vi "Main.vi"(11 "Module Admin":refnum<class "Delacor_lib_QMH_Module Admin.lvclass">) -> ()   [LabVIEW 2022 SP3, in "HW-201 Manager.lvlib"]
doc: "This template is based off of the Queued Message Handler design pattern and the Queued Message Handler project template that ships with LabVIEW.\n\nThe main difference is that the queue is private to this module and communication between modules is performed via Broadcast and Request events.\n\nRequest events are wrapped in public API methods and are handled in the Event Handling Loop (EHL) of this VI. Any module can register for Broadcast events sent by this module. The EHL generates messages based on user interface actions.\n\nThe Message Handling Loop (MHL) processes messages generated by the EHL, or by other messages. The messages are string values, so new messages can be added easily to the Message Cases case structure in the MHL. Each message cluster can also provide an optional value for Message Data, which is a variant that can be converted to whatever message-specific data is required.\n_____\nBased on DQMH Project Template 7.0.1.1316."
uses:
  HW-201 Manager.lvlib
  <vilib>/Delacor/Delacor QMH/Libraries/Module Admin_class/Delacor_lib_QMH_Module Admin.lvclass
  Module Data--cluster.ctl
  Do Something Argument--cluster.ctl
  <vilib>/Delacor/Delacor QMH/Libraries/Message Queue_class/Delacor_lib_QMH_Message Queue.lvclass/Delacor_lib_QMH_Message Queue.ctl
  Do Something Else Argument--cluster.ctl
  Do Something Else and Wait for Reply Argument--cluster.ctl
  Do Something Else and Wait (Reply Payload)--cluster.ctl
  Stop Argument--cluster.ctl
  <vilib>/Delacor/Delacor QMH/Libraries/Module Admin_class/Delacor_lib_QMH_Module Admin.lvclass/Delacor_lib_QMH_Module Admin.ctl
  <vilib>/Utility/miscctls.llb/LVPointTypeDef.ctl
  <vilib>/Delacor/Delacor QMH/Libraries/Message Queue_class/Delacor_lib_QMH_Enqueue Message (Single).vi
  <vilib>/Delacor/Delacor QMH/Libraries/Module Admin_class/Delacor_lib_QMH_Get External Launch.vi
  <vilib>/Delacor/Delacor QMH/Libraries/Message Queue_class/Delacor_lib_QMH_Message Queue.lvclass
panel:
  out "error out":errorcluster
  out "X":dbl
  out "Status":string
  in  "Simulate MHL Error":bool
  in  "Simulate EHL Error":bool
  in  "Do Something Else <Replace Me>":bool
  in  "Do Something <Replace Me>":bool
  # "These controls have associated \"Value Changed\" events configured in the Event Structure on the diagram.\n\nReplace them (and reconfigure the Event Structure) with the controls you need for your application. \n\nOther processes communicate with this Module via its Public API (wrappers for its Request Events).\n\nThis Module communicates with other processes via its Broadcast Events.\nAny process that wants to receive these messages can register for this module's Broadcast events."
  # "This template is for the DQMH framework. See the block diagram for more information on how to use this template."
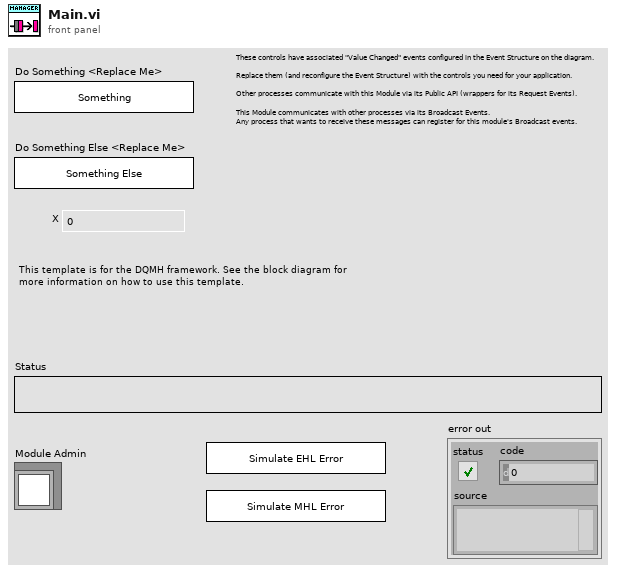
[diagram p1: front panel]
types:
  T1 = typedef "HW-201 Manager.lvlib/Request Events--cluster.ctl" = cluster{"Stop Module":refnum<user-event>, "Do Something":refnum<user-event>, "Do Something Else":refnum<user-event>, "Do Something Else and Wait for Reply":refnum<user-event>, "Show Panel":refnum<user-event>, "Hide Panel":refnum<user-event>, "Get Module Execution Status":refnum<user-event>, "Show Diagram":refnum<user-event>}
  T2 = typedef "HW-201 Manager.lvlib/Module Data--cluster.ctl" = cluster{"Status":string}
  T3 = typedef "HW-201 Manager.lvlib/Do Something Argument--cluster.ctl" = cluster{"Do Something Msg":string}
  T4 = typedef "HW-201 Manager.lvlib/Do Something Else Argument--cluster.ctl" = cluster{"Do Something Else Msg":string, "X":dbl}
  T5 = typedef "HW-201 Manager.lvlib/Do Something Else and Wait for Reply Argument--cluster.ctl" = cluster{"Do Something Else Msg":string, "X":dbl, "Wait Notifier":refnum<notifier>, "wait for reply":bool}
  T6 = enum32{"invalid lock state", "Not Locked", "Locked (No Password)", "Password-protected"}
  T7 = typedef "HW-201 Manager.lvlib/Stop Argument--cluster.ctl" = cluster{"Origin":string, "Exit via Stop Module Req?":bool, "Wait for Module to stop?":bool}
  T8 = typedef "LVPointTypeDef.ctl" = cluster{"Horizontal":i16, "Vertical":i16}
  T9 = enum32{"Invalid", "Standard", "Closed", "Hidden", "Minimized", "Maximized"}
  T10 = typedef "HW-201 Manager.lvlib/Do Something Else and Wait (Reply Payload)--cluster.ctl" = cluster{"Value":dbl, "error":errorcluster}
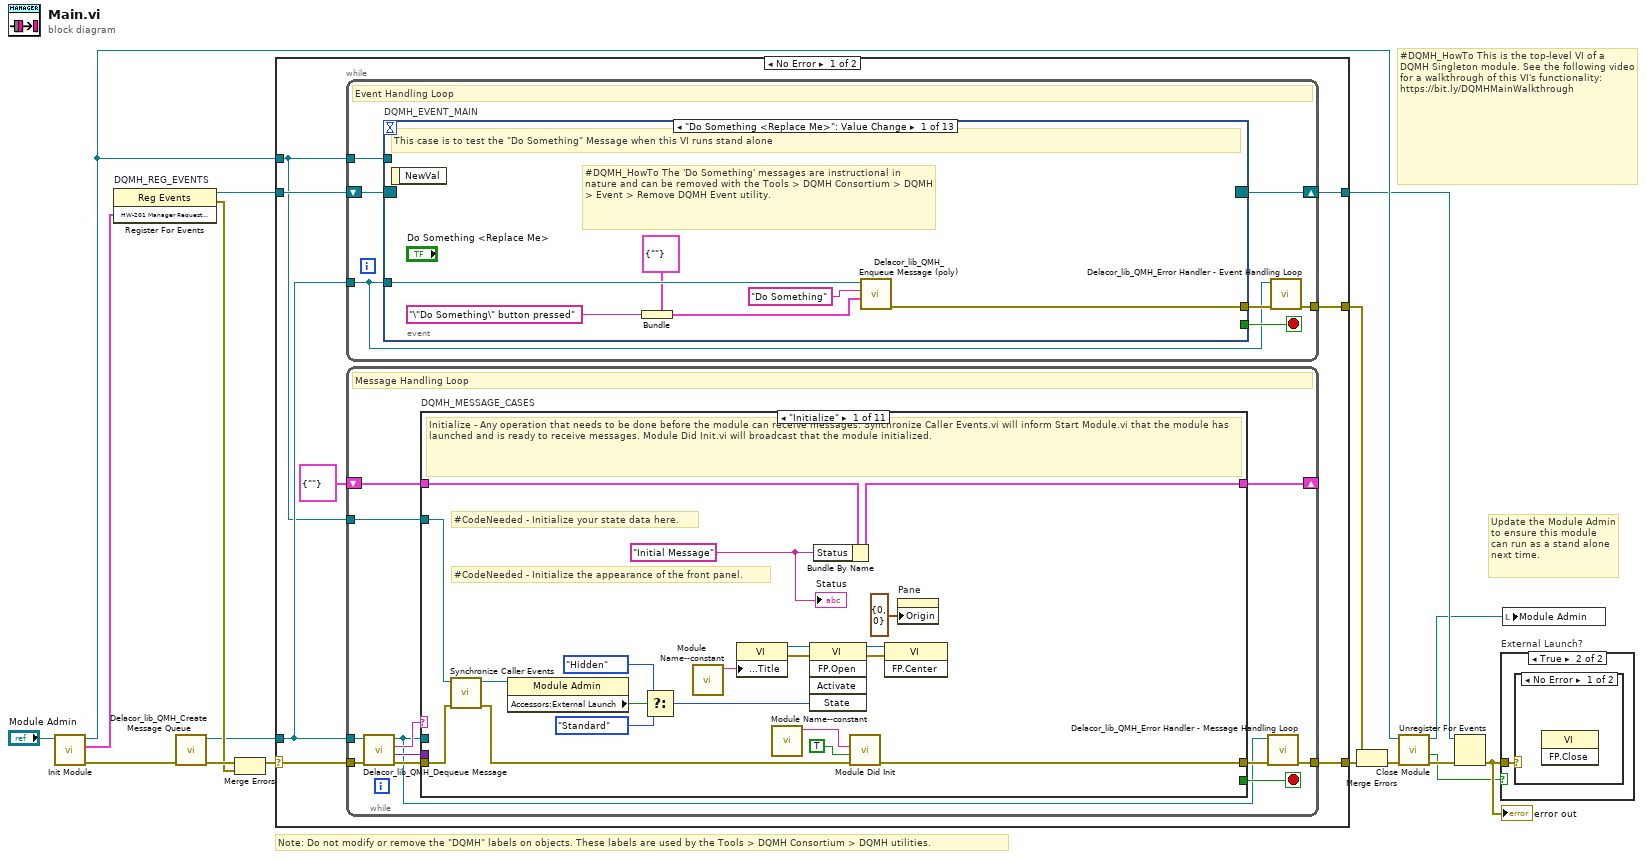
[diagram p0: block diagram]
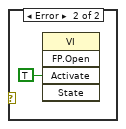
[diagram p3: hidden frame]
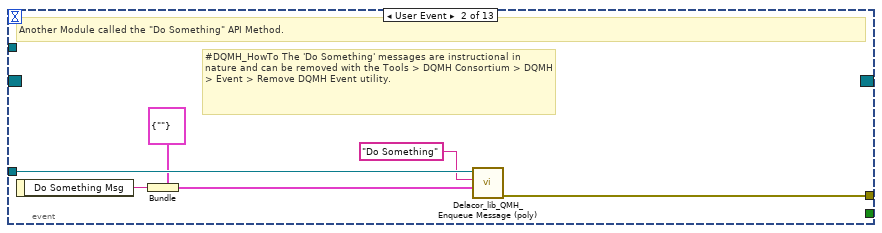
[diagram p4: hidden frame]
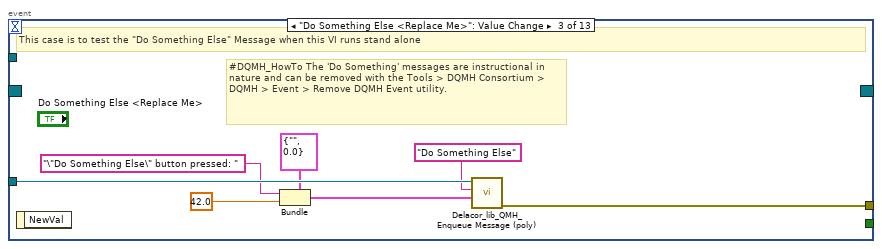
[diagram p5: hidden frame]
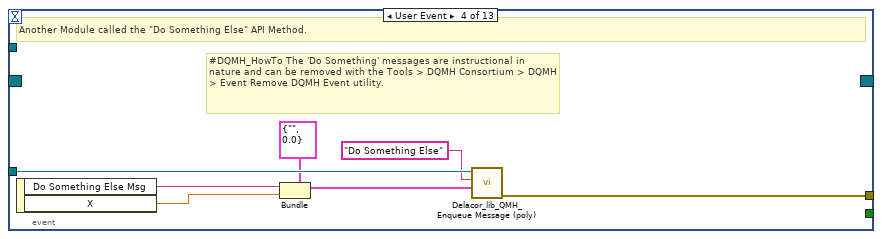
[diagram p6: hidden frame]
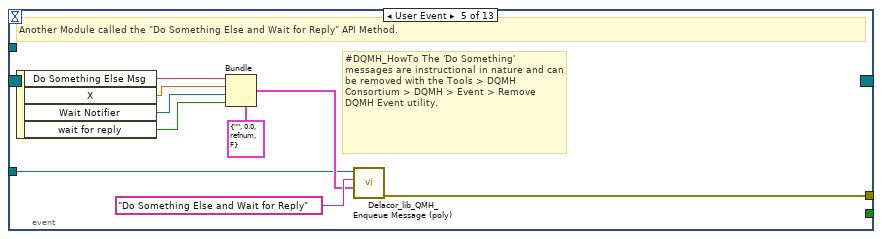
[diagram p7: hidden frame]
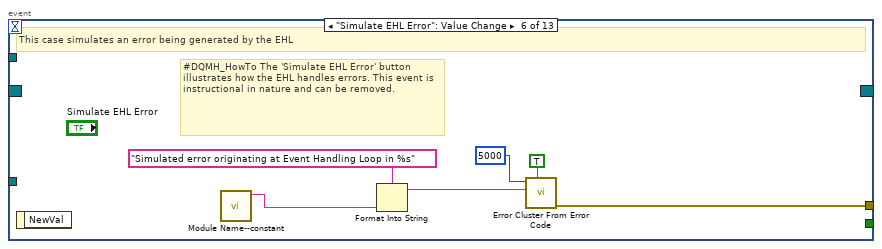
[diagram p8: hidden frame]
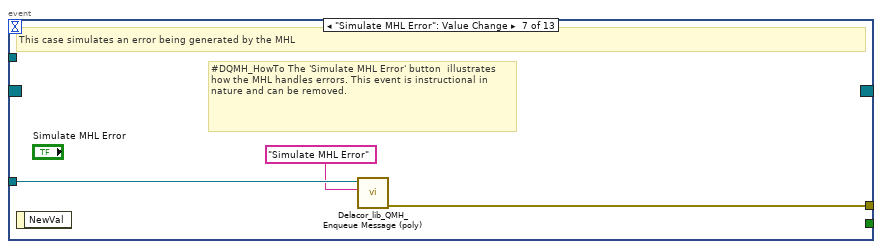
[diagram p9: hidden frame]
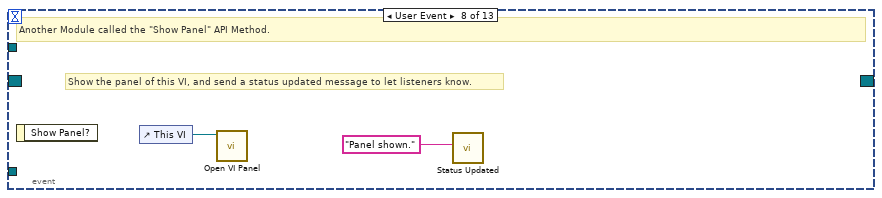
[diagram p10: hidden frame]
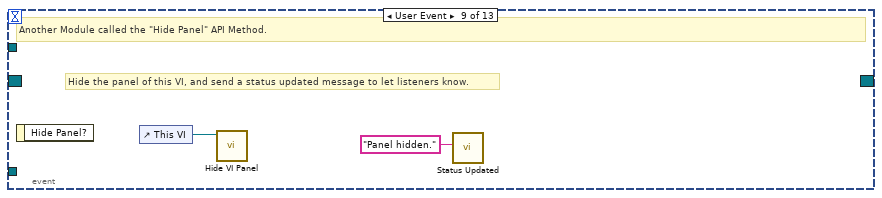
[diagram p11: hidden frame]
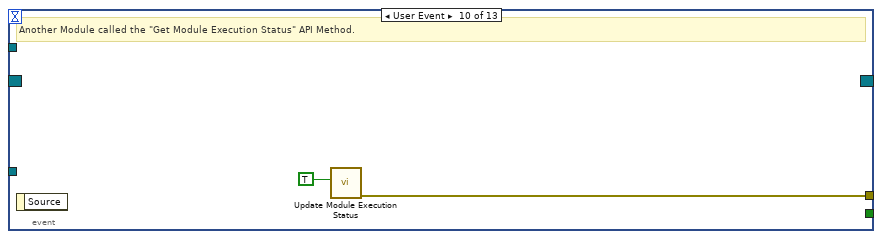
[diagram p12: hidden frame]
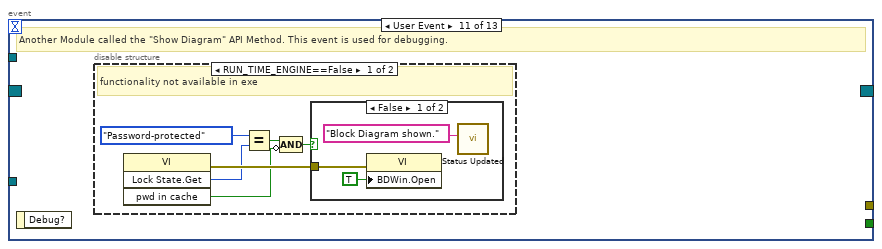
[diagram p13: hidden frame]
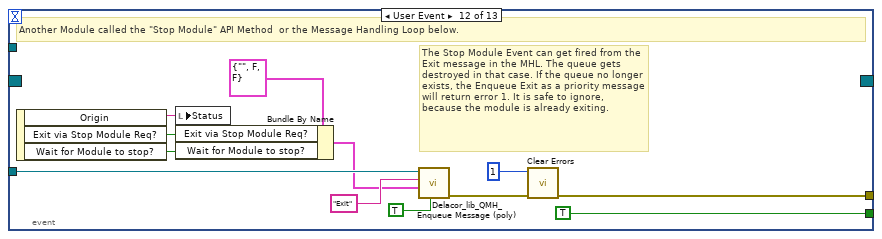
[diagram p16: hidden frame]
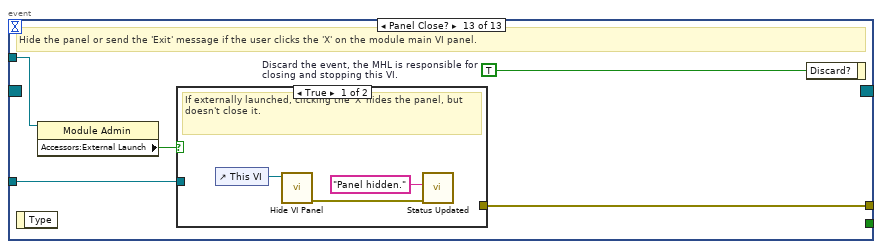
[diagram p17: hidden frame]
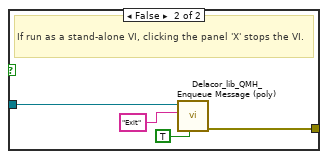
[diagram p18: hidden frame]
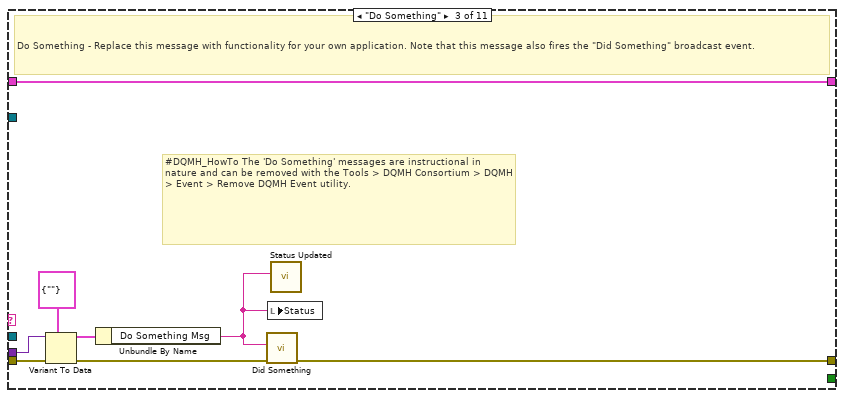
[diagram p20: hidden frame]
diagram:
  # "#DQMH_HowTo This is the top-level VI of a DQMH Singleton module. See the following video for a walkthrough of this VI's functionality: https://bit.ly/DQMHMainWalkthrough"
  # "Note: Do not modify or remove the \"DQMH\" labels on objects. These labels are used by the Tools > DQMH Consortium > DQMH utilities."
  # "Update the Module Admin to ensure this module can run as a stand alone next time."
  n1 = call "Init Module.vi"("Singleton Module Admin in"="Module Admin") -> ("error out"=w16:errorcluster, "HW-201 Manager Request Events"=w5:T1, "Singleton Module Admin out"=w8:refnum<class "Delacor_lib_QMH_Module Admin.lvclass">)  [unwired: 8 in]
  n2 = register-events "DQMH_REG_EVENTS"(w5) -> (reference out=w6:refnum<event-registration>, error out=w9:errorcluster)  [unwired: 2 in]
  n3 = call <vilib>:"Delacor_lib_QMH_Create Message Queue.vi"("error in"=w16) -> ("error out"=w11:errorcluster, "Message Queue"=w4:refnum<class "Delacor_lib_QMH_Message Queue.lvclass">)  [unwired: 9 in]
  n4 = Merge Errors(w11, w9) -> (w10:errorcluster)
  n5 = case shown="No Error" w10 {
    selector: w10 -> [w23 w259]
    tunnel: [w25 w258] -> w17
    tunnel: [w22 w257] -> w7
    tunnel: w6 -> [w20 w257]
    tunnel: w4 -> [w19 w252]
    tunnel: [w24 _] -> w14
    tunnel: w8 -> [w18 w253]
    frame No Error {
      n6 = while {
        tunnel: w19 -> [w26]
        shift-right: [w29] -> w22
        shift-left: w20 -> [w30]
        tunnel: [w31] -> w24
        tunnel: w18 -> [w27]
        stop <- w28 stop-if-true
        # "Event Handling Loop"
        n7 = event "DQMH_EVENT_MAIN" shown="[0] \"Do Something <Replace Me>\": Value Change" {
          selector: w30 -> [_ _ _ _ _ _ _ _ _ _ _ _ _]
          dyn-events: [_ _ _ _ _ _ _ _ _ _ _ _ _] -> w29
          timeout: _ -> [_ _ _ _ _ _ _ _ _ _ _ _ _]
          tunnel: [_ _ _ _ _ _ _ _ _ _ _ TRUE ("Discard?") _] -> w28
          tunnel: w26 -> [w37 w43 w50 w57 w60 _ w75 _ _ _ _ w99 w106]
          tunnel: [w38 w44 w51 w58 w67 w73 w76 _ _ w82 _ w102 w108] -> w32
          tunnel: w27 -> [_ _ _ _ _ _ _ _ _ _ _ _ w105]
          event "Do Something <Replace Me>": Value Change {
            # "#DQMH_HowTo The 'Do Something' messages are instructional in nature and can be removed with the Tools > DQMH Consortium > DQMH > Event > Remove DQMH Event utility."
            # "This case is to test the \"Do Something\" Message when this VI runs stand alone"
            n8 = event-data() -> ()  [unwired: 1 in, 1 out]
            n9 = Bundle(cluster=T3 {"Do Something Msg"=""} ("Do Something Argument"), "Do Something Msg"="\"Do Something\" button pressed" ("\"Do Something\" button pressed")) -> (w33:T3)
            n10 = call-poly <vilib>:"Delacor_lib_QMH_Enqueue Message (poly).vi"("Message Data"=w33, "Message"="Do Something", "Message Queue in"=w37) -> ("error out"=w38:errorcluster)  [unwired: 7 in, 1 out]
          }
          event User Event {
            # "#DQMH_HowTo The 'Do Something' messages are instructional in nature and can be removed with the Tools > DQMH Consortium > DQMH > Event > Remove DQMH Event utility."
            # "Another Module called the \"Do Something\" API Method."
            n11 = event-data() -> ("Do Something Msg"=w40:string)  [unwired: 1 in]
            n12 = Bundle(cluster=T3 {"Do Something Msg"=""} ("Do Something Argument"), "Do Something Msg"=w40) -> (w39:T3)
            n13 = call-poly <vilib>:"Delacor_lib_QMH_Enqueue Message (poly).vi"("Message Data"=w39, "Message"="Do Something", "Message Queue in"=w43) -> ("error out"=w44:errorcluster)  [unwired: 7 in, 1 out]
          }
          event "Do Something Else <Replace Me>": Value Change {
            # "#DQMH_HowTo The 'Do Something' messages are instructional in nature and can be removed with the Tools > DQMH Consortium > DQMH > Event > Remove DQMH Event utility."
            # "This case is to test the \"Do Something Else\" Message when this VI runs stand alone"
            n14 = event-data() -> ()  [unwired: 1 in, 1 out]
            n15 = Bundle(cluster=T4 {"Do Something Else Msg"="", "X"=0.0} ("Do Something Else Argument"), "Do Something Else Msg"="\"Do Something Else\" button pressed: " ("\"Do Something Else\" button pressed"), "X"=42.0) -> (w47:T4)
            n16 = call-poly <vilib>:"Delacor_lib_QMH_Enqueue Message (poly).vi"("Message Data"=w47, "Message"="Do Something Else", "Message Queue in"=w50) -> ("error out"=w51:errorcluster)  [unwired: 7 in, 1 out]
          }
          event User Event {
            # "#DQMH_HowTo The 'Do Something' messages are instructional in nature and can be removed with the Tools > DQMH Consortium > DQMH > Event Remove DQMH Event utility."
            # "Another Module called the \"Do Something Else\" API Method."
            n17 = event-data() -> ("Do Something Else Msg"=w53:string, "X"=w52:dbl)  [unwired: 1 in]
            n18 = Bundle(cluster=T4 {"Do Something Else Msg"="", "X"=0.0} ("Do Something Else Argument"), "Do Something Else Msg"=w53, "X"=w52) -> (w54:T4)
            n19 = call-poly <vilib>:"Delacor_lib_QMH_Enqueue Message (poly).vi"("Message Data"=w54, "Message"="Do Something Else", "Message Queue in"=w57) -> ("error out"=w58:errorcluster)  [unwired: 7 in, 1 out]
          }
          event User Event {
            # "#DQMH_HowTo The 'Do Something' messages are instructional in nature and can be removed with the Tools > DQMH Consortium > DQMH > Event > Remove DQMH Event utility."
            # "Another Module called the \"Do Something Else and Wait for Reply\" API Method."
            n20 = event-data() -> ("Do Something Else Msg"=w63:string, "X"=w62:dbl, "Wait Notifier"=w61:refnum<notifier>, "wait for reply"=w59:bool)  [unwired: 1 in]
            n21 = Bundle(cluster=T5 {"Do Something Else Msg"="", "X"=0.0, "Wait Notifier"=refnum, "wait for reply"=FALSE} ("Do Something Else and Wait for Reply Argument"), "Do Something Else Msg"=w63, "X"=w62, "Wait Notifier"=w61, "wait for reply"=w59) -> (w64:T5)
            n22 = call-poly <vilib>:"Delacor_lib_QMH_Enqueue Message (poly).vi"("Message Data"=w64, "Message"="Do Something Else and Wait for Reply", "Message Queue in"=w60) -> ("error out"=w67:errorcluster)  [unwired: 7 in, 1 out]
          }
          event "Simulate EHL Error": Value Change {
            # "#DQMH_HowTo The 'Simulate EHL Error' button  illustrates how the EHL handles errors. This event is instructional in nature and can be removed."
            # "This case simulates an error being generated by the EHL"
            n23 = event-data() -> ()  [unwired: 1 in, 1 out]
            n24 = call "Module Name--constant.vi"() -> ("Module Name"=w70:string)  [unwired: 11 in]
            n25 = Format Into String(format string="Simulated error originating at Event Handling Loop in %s", w70) -> (resulting string=w71:string)  [unwired: 2 in, 1 out]
            n26 = call <vilib>:"Error Cluster From Error Code.vi"("show call chain? (False)"=TRUE, "error message (\"\")"=w71, "error code (0)"=5000) -> ("error out"=w73:errorcluster)  [unwired: 6 in]
          }
          event "Simulate MHL Error": Value Change {
            # "#DQMH_HowTo The 'Simulate MHL Error' button  illustrates how the MHL handles errors. This event is instructional in nature and can be removed."
            # "This case simulates an error being generated by the MHL"
            n27 = event-data() -> ()  [unwired: 1 in, 1 out]
            n28 = call-poly <vilib>:"Delacor_lib_QMH_Enqueue Message (poly).vi"("Message"="Simulate MHL Error", "Message Queue in"=w75) -> ("error out"=w76:errorcluster)  [unwired: 8 in, 1 out]
          }
          event User Event {
            # "Show the panel of this VI, and send a status updated message to let listeners know."
            # "Another Module called the \"Show Panel\" API Method."
            n29 = event-data() -> ()  [unwired: 1 in, 1 out]
            n30 = control-ref of="This VI"() -> (w78:refnum<vi>)
            n31 = call "Open VI Panel.vi"("VI"=w78) -> ()  [unwired: 10 in, 1 out]
            n32 = call "Status Updated.vi"("Status"="Panel shown." ("format string")) -> ()  [unwired: 10 in, 1 out]
          }
          event User Event {
            # "Hide the panel of this VI, and send a status updated message to let listeners know."
            # "Another Module called the \"Hide Panel\" API Method."
            n33 = event-data() -> ()  [unwired: 1 in, 1 out]
            n34 = control-ref of="This VI"() -> (w80:refnum<vi>)
            n35 = call "Hide VI Panel.vi"("VI"=w80) -> ()  [unwired: 10 in, 1 out]
            n36 = call "Status Updated.vi"("Status"="Panel hidden." ("format string")) -> ()  [unwired: 10 in, 1 out]
          }
          event User Event {
            # "Another Module called the \"Get Module Execution Status\" API Method."
            n37 = event-data() -> ()  [unwired: 1 in, 1 out]
            n38 = call "Update Module Execution Status.vi"("Running?"=TRUE) -> ("error out"=w82:errorcluster)  [unwired: 10 in]
          }
          event User Event {
            # "Another Module called the \"Show Diagram\" API Method. This event is used for debugging."
            n39 = event-data() -> ()  [unwired: 1 in, 1 out]
            n40 = disable-structure shown="RUN_TIME_ENGINE==False" {
              frame condition #0 (active) {
                # "functionality not available in exe"
                n41 = invoke on="Invoke Node" class="VI" method="Lock State.Get"() -> (error out=w88:errorcluster, "Get Lock State"=w87:T6, "pwd in cache"=w84:bool)  [unwired: 4 in, 1 out]
                n42 = Equal?(x=T6."Password-protected", y=w87) -> (x = y?=w85:bool)
                n43 = Compound Arithmetic op=AND(w85, invert w84) -> (w83:bool)
                n44 = case shown="False" w83 {
                  tunnel: w88 -> [w91 _]
                  frame False {
                    n45 = property on="Property Node" class="VI"(error in=w91, "BDWin.Open"=TRUE ("Block Diagram Window:Open")) -> ()  [unwired: 1 in, 2 out]
                    n46 = call "Status Updated.vi"("Status"="Block Diagram shown." ("format string")) -> ()  [unwired: 10 in, 1 out]
                  }
                  frame True {
                    # "Password-protected VI, and the password is not in the cache. Do not show the diagram."
                  }
                }
              }
              frame condition #1 {
              }
            }
          }
          event User Event {
            # "The Stop Module Event can get fired from the Exit message in the MHL. The queue gets destroyed in that case. If the queue no longer exists, the Enqueue Exit as a priority message will return error 1. It is safe to ignore, because the module is already exiting."
            # "Another Module called the \"Stop Module\" API Method  or the Message Handling Loop below."
            n47 = event-data() -> ("Origin"=w98:string, "Exit via Stop Module Req?"=w94:bool, "Wait for Module to stop?"=w93:bool)  [unwired: 1 in]
            n48 = local write "Status"(w98) -> ()
            n49 = Bundle By Name(cluster=T7 {"Origin"="", "Exit via Stop Module Req?"=FALSE, "Wait for Module to stop?"=FALSE} ("Stop Argument"), "Exit via Stop Module Req?"=w94, "Wait for Module to stop?"=w93) -> (w92:T7)
            n50 = call-poly <vilib>:"Delacor_lib_QMH_Enqueue Message (poly).vi"("Priority Message? (F)"=TRUE, "Message Data"=w92, "Message"="Exit", "Message Queue in"=w99) -> ("error out"=w103:errorcluster)  [unwired: 6 in, 1 out]
            n51 = call <vilib>:"Clear Errors.vi"("error in (no error)"=w103, "specific error code to clear (0: all)"=1) -> ("error out"=w102:errorcluster)  [unwired: 4 in, 1 out]
          }
          event Panel Close? {
            w107 = TRUE  # Discard the event, the MHL is responsible for closing and stopping this VI.
            # "Hide the panel or send the 'Exit' message if the user clicks the 'X' on the module main VI panel."
            n52 = event-data() -> ()  [unwired: 1 in, 1 out]
            n53 = property on="Property Node" class="Module Admin"(reference=w105) -> ("Accessors:External Launch"=w104:bool)  [unwired: 1 in, 2 out]
            n54 = case shown="True" w104 {
              tunnel: w106 -> [_ w114]
              tunnel: [_ w115] -> w108
              frame True {
                # "If externally launched, clicking the 'X' hides the panel, but doesn't close it."
                n55 = control-ref of="This VI"() -> (w111:refnum<vi>)
                n56 = call "Hide VI Panel.vi"("VI"=w111) -> ("error out"=w109:errorcluster)  [unwired: 10 in]
                n57 = call "Status Updated.vi"("error in"=w109, "Status"="Panel hidden." ("format string")) -> ()  [unwired: 9 in, 1 out]
              }
              frame False {
                # "If run as a stand-alone VI, clicking the panel 'X' stops the VI."
                n58 = call-poly <vilib>:"Delacor_lib_QMH_Enqueue Message (poly).vi"("Priority Message? (F)"=TRUE, "Message"="Exit", "Message Queue in"=w114) -> ("error out"=w115:errorcluster)  [unwired: 7 in, 1 out]
              }
            }
            n59 = event-data ("Event Filter Node")("Discard?"=w107) -> ()  [unwired: 1 in, 1 out]
          }
        }
        n60 = call-dynamic "Delacor_lib_QMH_Error Handler - Event Handling Loop.vi"("error in"=w32, "Message Queue in"=w26) -> ("dup error in"=w31:errorcluster)  [unwired: 8 in, 1 out]
      }
      n61 = while {
        tunnel: w19 -> [w116]
        shift-right: [w124] -> _
        shift-left: T2 {"Status"=""} ("Data Cluster") -> [w125]
        tunnel: w23 -> [w127]
        tunnel: [w119] -> w25
        tunnel: w18 -> [w120]
        stop <- w123 stop-if-true
        # "Message Handling Loop"
        n62 = call-dynamic "Delacor_lib_QMH_Dequeue Message.vi"("error in"=w127, "Message Queue in"=w116) -> ("error out"=w126:errorcluster, "Message Data"=w121:variant, "Message"=w122:string, "Message Queue out"=w117:refnum<class "Delacor_lib_QMH_Message Queue.lvclass">)  [unwired: 6 in]
        n63 = case "DQMH_MESSAGE_CASES" shown="\"Initialize\"" w122 {
          selector: w122 -> [_ _ _ _ _ _ _ _ _ _ w247]
          tunnel: w117 -> [_ _ _ _ _ _ _ _ w213 w235 _]
          tunnel: w126 -> [w145 w149 w157 w166 w185 w198 w200 w209 w220 w241 w250]
          tunnel: [w143 w149 w155 w165 w184 w197 w200 w208 w216 w236 w251] -> w118
          tunnel: w125 -> [w134 w148 w154 w164 w181 w196 w199 w206 w215 w234 w248]
          tunnel: [w133 w148 w154 w164 w181 w196 w199 w206 w215 w234 w248] -> w124
          tunnel: [_ _ _ _ _ _ _ _ _ w233 _] -> w123
          tunnel: w121 -> [_ _ w153 w161 w178 _ _ _ w214 w232 _]
          tunnel: w120 -> [w135 _ _ _ _ _ _ _ w212 w227 _]
          frame "Initialize" {
            w129 = "Initial Message" ("Initial Message")
            # "#CodeNeeded - Initialize the appearance of the front panel."
            # "#CodeNeeded - Initialize your state data here."
            # "Initialize - Any operation that needs to be done before the module can receive messages. Synchronize Caller Events.vi will inform Start Module.vi that the module has launched and is ready to receive messages. Module Did Init.vi will broadcast that the module initialized."
            n64 = call "Synchronize Caller Events.vi"("error in"=w145, "Singleton Module Admin in"=w135) -> ("error out"=w144:errorcluster, "Singleton Module Admin out"=w130:refnum<class "Delacor_lib_QMH_Module Admin.lvclass">)  [unwired: 8 in]
            n65 = property on="Property Node" class="Module Admin"(reference=w130) -> ("Accessors:External Launch"=w139:bool)  [unwired: 1 in, 2 out]
            n66 = Select(t=T9."Hidden" ("State"), s=w139, f=T9."Standard" ("State")) -> (s? t:f=w136:T9)
            n67 = call "Module Name--constant.vi"() -> ("Module Name"=w142:string)  [unwired: 11 in]
            n68 = property on="Property Node" class="VI"("Front Panel.Title"=w142) -> (reference out=w141:refnum<vi>, error out=w147:errorcluster)  [unwired: 2 in]
            n69 = call "Module Name--constant.vi"() -> ("Module Name"=w131:string)  [unwired: 11 in]
            n70 = invoke on="Invoke Node" class="VI" method="FP.Open"(reference=w141, error in=w147, "State"=w136) -> (reference out=w140:refnum<vi>, error out=w146:errorcluster)  [unwired: 2 in, 3 out]
            n71 = Bundle By Name(cluster=w134, "Status"=w129) -> (w133:T2)
            n72 = call "Module Did Init.vi"("error in"=w144, "Initialized?"=TRUE, "Origin"=w131) -> ("error out"=w143:errorcluster)  [unwired: 8 in]
            n73 = invoke on="Invoke Node" class="VI" method="FP.Center"(reference=w140, error in=w146) -> ()  [unwired: 1 in, 3 out]
            n74 = property on="Pane" class="Pane"("Origin"=T8 {"Horizontal"=0, "Vertical"=0}) -> ()  [unwired: 2 in, 2 out]
            "Status" <- w129
          }
          frame "---Module Specific---" {
            # "Separator -- The following cases handle messages specific to this Module."
          }
          frame "Do Something" {
            # "#DQMH_HowTo The 'Do Something' messages are instructional in nature and can be removed with the Tools > DQMH Consortium > DQMH > Event > Remove DQMH Event utility."
            # "Do Something - Replace this message with functionality for your own application. Note that this message also fires the \"Did Something\" broadcast event."
            n75 = Variant To Data(error in=w157, type=T3 {"Do Something Msg"=""} ("Do Something Argument"), Variant=w153) -> (data=w152:T3, error out=w156:errorcluster)
            n76 = Unbundle By Name(w152) -> ("Do Something Msg"=w150:string)
            n77 = call "Did Something.vi"("error in"=w156, "Did Something Msg"=w150) -> ("error out"=w155:errorcluster)  [unwired: 9 in]
            n78 = local write "Status"(w150) -> ()
            n79 = call "Status Updated.vi"("Status"=w150) -> ()  [unwired: 10 in, 1 out]
          }
          frame "Do Something Else" {
            # "#DQMH_HowTo The 'Do Something' messages are instructional in nature and can be removed with the Tools > DQMH Consortium > DQMH > Event > Remove DQMH Event utility."
            # "Do Something Else - Replace this message with functionality for your own application."
            n80 = Variant To Data(error in=w166, type=T4 {"Do Something Else Msg"="", "X"=0.0} ("Do Something Else Argument"), Variant=w161) -> (data=w162:T4, error out=w165:errorcluster)
            n81 = Unbundle By Name(w162) -> ("Do Something Else Msg"=w160:string, "X"=w159:dbl)
            "X" <- w159
            n82 = Format Into String(initial string=w160, w159) -> (resulting string=w158:string)  [unwired: 2 in, 1 out]
            n83 = local write "Status"(w158) -> ()
            n84 = call "Status Updated.vi"("Status"=w158) -> ()  [unwired: 10 in, 1 out]
          }
          frame "Do Something Else and Wait for Reply" {
            w173 = "X(%.2f)+Offset(%.2f)=%.2f"  # status message format string
            # "#DQMH_HowTo The 'Do Something' messages are instructional in nature and can be removed."
            # "Send back X with a random offset"
            # "Do Something Else and Wait for Reply - Replace this message with functionality for your own application. Note that this message must fire a notifier to let callers know it has finished execution, and it returns an error if the 'Value' is negative."
            n85 = Variant To Data(error in=w185, type=T5 {"Do Something Else Msg"="", "X"=0.0, "Wait Notifier"=refnum, "wait for reply"=FALSE} ("Do Something Else and Wait for Reply Argument"), Variant=w178) -> (data=w179:T5, error out=w183:errorcluster)
            n86 = Unbundle By Name(w179) -> ("Wait Notifier"=w167:refnum<notifier>, "Do Something Else Msg"=w177:string, "X"=w174:dbl, "wait for reply"=w170:bool)
            n87 = Random Number (0-1)() -> (number: 0 to 1=w175:dbl)
            n88 = Add(x=w175, y=w174) -> (x+y=w169:dbl)
            n89 = Less Than 0?(x=w169) -> (x < 0?=w172:bool)
            n90 = local write "X"(w174) -> ()
            n91 = case shown="True" w172 {
              tunnel: [_ w195] -> w182
              frame False {
              }
              frame True {
                n92 = call <vilib>:"Error Cluster From Error Code.vi"("show call chain? (False)"=TRUE, "error message (\"\")"="The 'Something Else and Wait for Reply' message generated a negative number, which is considered an error condition.", "error code (0)"=5000) -> ("error out"=w195:errorcluster)  [unwired: 6 in]
              }
            }
            n93 = Format Into String(format string=w173, initial string=w177, w174, w175, w169) -> (resulting string=w171:string)  [unwired: 1 in, 1 out]
            n94 = Bundle By Name(cluster=T10 {"Value"=0.0, "error"={"status"=FALSE, "code"=0, "source"=""}} ("notification"), "error"=w182, "Value"=w169) -> (w168:T10)
            n95 = local write "Status"(w171) -> ()
            n96 = call "Status Updated.vi"("Status"=w171) -> ()  [unwired: 10 in, 1 out]
            n97 = case shown="True" w170 {
              tunnel: w168 -> [_ w188]
              tunnel: w167 -> [_ w187]
              frame False {
              }
              frame True {
                # "Simulate an operation that requires a wait."
                n98 = flat-sequence {
                  tunnel: w188 -> [w191]
                  tunnel: w187 -> [w190]
                  tunnel: w186 -> [_]
                  frame #0 {
                    n99 = Send Notification(notification=w191, notifier=w190) -> ()  [unwired: 1 in, 2 out]
                  }
                }
                n100 = Wait (ms)(milliseconds to wait=u32 1000) -> (millisecond timer value=w186:u32)
              }
            }
            n101 = Merge Errors(w183, w182) -> (w184:errorcluster)
          }
          frame "---Copy This Frame---" {
            # "Duplicate this frame when creating new messages.  Change this comment in the duplicated frame to describe this message."
            n102 = Merge Errors(w198) -> (w197:errorcluster)
          }
          frame "---Exit and Error Handling---" {
            # "Separator - The following cases handle errors and exit messages."
          }
          frame "Simulate MHL Error" {
            # "#DQMH_HowTo The 'Simulate MHL Error' button  illustrates how the MHL handles errors. This event is instructional in nature and can be removed."
            # "Simulate an error occurring at the MHL"
            n103 = call "Module Name--constant.vi"() -> ("Module Name"=w202:string)  [unwired: 11 in]
            n104 = Format Into String(format string="Simulated error originating at Message Handling Loop in %s", w202) -> (resulting string=w203:string)  [unwired: 2 in, 1 out]
            n105 = call <vilib>:"Error Cluster From Error Code.vi"("show call chain? (False)"=TRUE, "error message (\"\")"=w203, "error code (0)"=5001) -> ("error out"=w207:errorcluster)  [unwired: 6 in]
            n106 = Merge Errors(w209, w207) -> (w208:errorcluster)
          }
          frame "Error" {
            # "#CodeRecommended - If the module is running in standalone mode (External Launch = FALSE), this code will pop up an error dialog and call the 'Exit' message if an error occurs. Add more fine-grained error management here."
            # "Error - Check the error message data and respond accordingly. This message is sent by the \"Error Handler\" VIs at the end of each loop in this application."
            n107 = property on="Property Node" class="Module Admin"(reference=w212) -> ("Accessors:External Launch"=w211:bool)  [unwired: 1 in, 2 out]
            n108 = Variant To Data(error in=w220, type=errorcluster {"status"=FALSE, "code"=0, "source"=""} ("error constant"), Variant=w214) -> (data=w210:errorcluster, error out=w218:errorcluster)
            n109 = local write "error out"(w210) -> ()
            n110 = call "Error Reported.vi"("Error"=w210) -> ()  [unwired: 10 in, 1 out]
            n111 = case shown="False" w211 {
              tunnel: [w225 _] -> w217
              tunnel: w213 -> [w223 _]
              tunnel: w210 -> [w224 _]
              frame False {
                n112 = disable-structure shown="Default" {
                  disable-tunnel: w224 -> [w226 _]
                  frame condition #0 (active) {
                    # "If the module is running standalone, then pop up an error dialog and call the \"Exit\" message."
                    n113 = call <vilib>:"Simple Error Handler.vi"("error in (no error)"=w226) -> ()  [unwired: 4 in, 5 out]
                  }
                  frame condition #1 {
                    # "To prevent the Simple Error Handler VI from being loaded (e.g. when deploying to a Real-Time target), add the Conditional Disable Symbol \"DQMH_Disable_SEH\" to your project and set it to TRUE."
                  }
                }
                n114 = call-poly <vilib>:"Delacor_lib_QMH_Enqueue Message (poly).vi"("Priority Message? (F)"=TRUE, "Message"="Exit", "Message Queue in"=w223) -> ("error out"=w225:errorcluster)  [unwired: 7 in, 1 out]
              }
              frame True {
                # "If the module was launched externally, calling the Error Reported broadcast VI is the only action performed by the \"Error\" message. The module's caller can then process the error appropriately."
              }
            }
            n115 = Merge Errors(w218, w217) -> (w216:errorcluster)
          }
          frame "Exit" {
            w231 = 91  # 91: not all Exit messages will have an argument
            w233 = TRUE  # Stop the VI
            # "Release the message queue reference"
            # "#CodeNeeded - Add any required cleanup code here."
            # "Exit - Exit the application."
            n116 = Variant To Data(error in=w241, type=T7 {"Origin"="", "Exit via Stop Module Req?"=FALSE, "Wait for Module to stop?"=FALSE} ("Stop Argument"), Variant=w232) -> (data=w229:T7, error out=w238:errorcluster)
            n117 = call <vilib>:"Clear Errors.vi"("error in (no error)"=w238, "specific error code to clear (0: all)"=w231) -> ("error out"=w240:errorcluster)  [unwired: 4 in, 1 out]
            n118 = control-ref of="This VI"() -> (w228:refnum<vi>)
            n119 = call-dynamic "Delacor_lib_QMH_Release Message Queue.vi"("error in"=w240, "Message Queue"=w235) -> ("error out"=w239:errorcluster)  [unwired: 9 in]
            n120 = call "Handle Exit.vi"("Stop Argument"=w229, "Admin in"=w227, "VI reference"=w228) -> ("error out"=w237:errorcluster)  [unwired: 7 in, 1 out]
            n121 = Merge Errors(w239, w237) -> (w236:errorcluster)
            n122 = call "Error Reported.vi"("Error"=w236) -> ()  [unwired: 10 in, 1 out]
          }
          frame Default {
            # "'Default' case only runs if there is a message that isn't defined in any of the other cases.  Output a programming error."
            n123 = call "Module Name--constant.vi"() -> ("Module Name"=w246:string)  [unwired: 11 in]
            n124 = Format Into String(format string="The invalid message string \"%s\" was received in the Message Handling Loop for module \"%s\".", w247, w246) -> (resulting string=w242:string)  [unwired: 2 in, 1 out]
            n125 = call <vilib>:"Error Cluster From Error Code.vi"("show call chain? (False)"=TRUE, "error message (\"\")"=w242, "error code (0)"=1) -> ("error out"=w249:errorcluster)  [unwired: 6 in]
            n126 = Merge Errors(w250, w249) -> (w251:errorcluster)
          }
        }
        n127 = call-dynamic "Delacor_lib_QMH_Error Handler - Message Handling Loop.vi"("error in"=w118, "Message Queue in"=w117) -> ("dup error in"=w119:errorcluster)  [unwired: 8 in, 1 out]
      }
    }
    frame Error {
      # "Synchronize Caller Events.vi will inform Start Module.vi that the module has launched and will let the code calling Start Module.vi register for broadcasts and would permit the caller receive the broadcast that an error occurred at launch time."
      n128 = call-dynamic "Delacor_lib_QMH_Release Message Queue.vi"("error in"=w259, "Message Queue"=w252) -> ("error out"=w258:errorcluster)  [unwired: 9 in]
      n129 = call "Synchronize Caller Events.vi"("Singleton Module Admin in"=w253) -> ("error out"=w260:errorcluster)  [unwired: 9 in, 1 out]
      n130 = call "Module Name--constant.vi"() -> ("Module Name"=w256:string)  [unwired: 11 in]
      n131 = Format Into String(format string="An error occurred during initialization. %s is no longer running.", w256) -> (resulting string=w254:string)  [unwired: 2 in, 1 out]
      n132 = Merge Errors(w258, w260) -> (w261:errorcluster)
      n133 = call "Error Reported.vi"("Additional Information"=w254, "Error"=w261) -> ()  [unwired: 9 in, 1 out]
    }
  }
  n134 = Merge Errors(w14, w17) -> (w13:errorcluster)
  n135 = call "Close Module.vi"("error in"=w13, "Module Admin in"=w8) -> ("error out"=w15:errorcluster, "External Launch"=w1:bool, "Module Admin out"=w2:refnum<class "Delacor_lib_QMH_Module Admin.lvclass">)  [unwired: 7 in]
  n136 = Unregister For Events(event registration refnum=w7, error in=w15) -> (error out=w12:errorcluster)
  "error out" <- w12
  n137 = case "External Launch?" shown="True" w1 {
    tunnel: w12 -> [_ w262]
    frame False {
    }
    frame True {
      n138 = case shown="No Error" w262 {
        frame No Error {
          n139 = invoke on="Invoke Node" class="VI" method="FP.Close"() -> ()  [unwired: 3 in, 3 out]
        }
        frame Error {
          n140 = invoke on="Invoke Node" class="VI" method="FP.Open"("Activate"=TRUE ("Activate?")) -> ()  [unwired: 4 in, 5 out]
        }
      }
    }
  }
  n141 = local write "Module Admin"(w2) -> ()
